vi "irradiance 1030_global variable.vi"() -> ()   [LabVIEW 2021]
panel:
  out "irradiance 1030":dbl
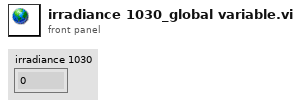
[diagram p1: front panel]
diagram:
